vi "PWM_Motor_Folgen.vi"(0 "Sensor gerade rechts":dbl=84.56879645320117, 1 "Sensor gerade links":dbl=69.1332619017031, 2 "Sensor schräg rechts":dbl=150.0, 3 "Sensor schräg links":dbl=54.38335596968736) -> (7 "PWM Motor":dbl=1.0)   [LabVIEW 2016]
uses:
  <vilib>/addons/control/pid/pid.llb/PID (DBL).vi
  <vilib>/addons/control/pid/NI_PID_pid.lvlib
panel:
  out "Waveform Chart":dbl(graph)
  in  "Array":dbl[](array[numeric])=[0.0, 0.0, 0.0, 0.0]
  in  "PID gains":T1={"proportional gain (Kc)"=-1.0, "integral time (Ti, min)"=0.01, "derivative time (Td, min)"=0.001} {"derivative time (Td, min)" format="%.3f"; "integral time (Ti, min)" format="%.3f"; "proportional gain (Kc)" format="%.3f"}
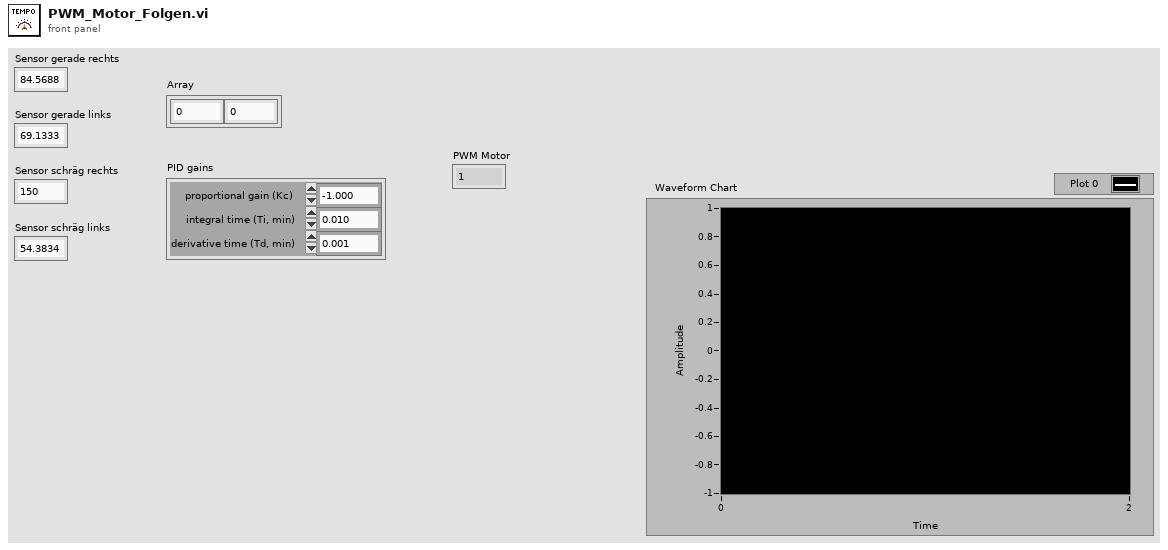
[diagram p1: front panel]
types:
  T1 = cluster{"proportional gain (Kc)":dbl, "integral time (Ti, min)":dbl, "derivative time (Td, min)":dbl}
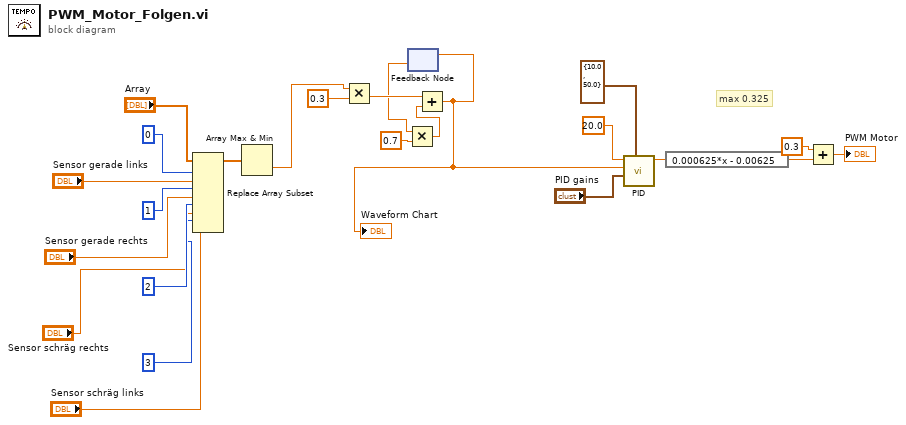
[diagram p0: block diagram]
diagram:
  # "max 0.325"
  n1 = Replace Array Subset(array="Array", new element #1="Sensor gerade links", index #1=0 ("index"), new element #2="Sensor gerade rechts", index #2=1 ("index"), new element #3="Sensor schräg rechts", index #3=2 ("index"), new element #4="Sensor schräg links", index #4=3 ("index")) -> (w5:dbl[])
  n2 = Array Max & Min(array=w5) -> (min value=w8:dbl)  [unwired: 3 out]
  n3 = Multiply(x=w8, y=0.3) -> (x*y=w11:dbl)
  n4 = feedback #1() -> (w9:dbl)  [unwired: 1 in]
  n5 = Multiply(x=w9, y=0.7) -> (x*y=w10:dbl)
  n6 = Add(x=w11, y=w10) -> (x+y=w7:dbl)
  "Waveform Chart" <- w7
  n7 = feedback-in #1(w7) -> ()
  n8 = call-poly <vilib>:"PID.vi"("output range"=cluster{"output high":dbl, "output low":dbl} {"output high"=10.0, "output low"=50.0}, "PID gains"="PID gains", "process variable"=w7, "setpoint"=20.0) -> ("output"=w16:dbl)  [unwired: 6 in, 1 out]
  n9 = expression code="0.000625*x - 0.00625"(w16) -> (w15:dbl)
  n10 = Add(x=0.3, y=w15) -> (x+y=→"PWM Motor":dbl)
